vi "StopProcess.Do.vi"(8 "error in":errorcluster, 10 "State Variables":T5, 11 "gRPC Request":T1) -> (0 "error out":errorcluster, 2 "State Variables out":T5, 3 "gRPC Response":T3)   [LabVIEW 2025, in "bus_monitor_server_do.lvlib"]
doc: "Stop all XNET sessions (Incoming and Outgoing).\nStop Async StreamProcess.Main.vi."
uses:
  bus_monitor_server_do.lvlib
  bus_monitor_server/RPC Messages/ni_bus_monitor_api_StopProcessReply.ctl
  bus_monitor_server/bus_monitor_server.lvlib
  bus_monitor_server/RPC Messages/ni_bus_monitor_api_ErrorInfo.ctl
  Types/XNET.InitialSettings.ctl
  Types/StreamProcess.VIRef.ctl
  Types/StreamProcess.Refs.ctl
  Types/MainProcess.StateVariables.ctl
  bus_monitor_server/RPC Messages/ni_bus_monitor_api_StopProcessRequest.ctl
  bus_monitor_server/RPC Messages/ni_bus_monitor_api_Session.ctl
  bus_monitor_server/RPC Messages/ni_bus_monitor_api_FrameFilter.ctl
  bus_monitor_server/RPC Messages/ni_bus_monitor_api_DirectionFilter.ctl
  bus_monitor_server/RPC Messages/ni_bus_monitor_api_FilterInfo.ctl
  bus_monitor_server/RPC Messages/ni_bus_monitor_api_FdIsoMode.ctl
  bus_monitor_server/RPC Messages/ni_bus_monitor_api_Termination.ctl
  bus_monitor_server/RPC Messages/ni_bus_monitor_api_CanMode.ctl
  bus_monitor_server/RPC Messages/ni_bus_monitor_api_ConnectSettings.ctl
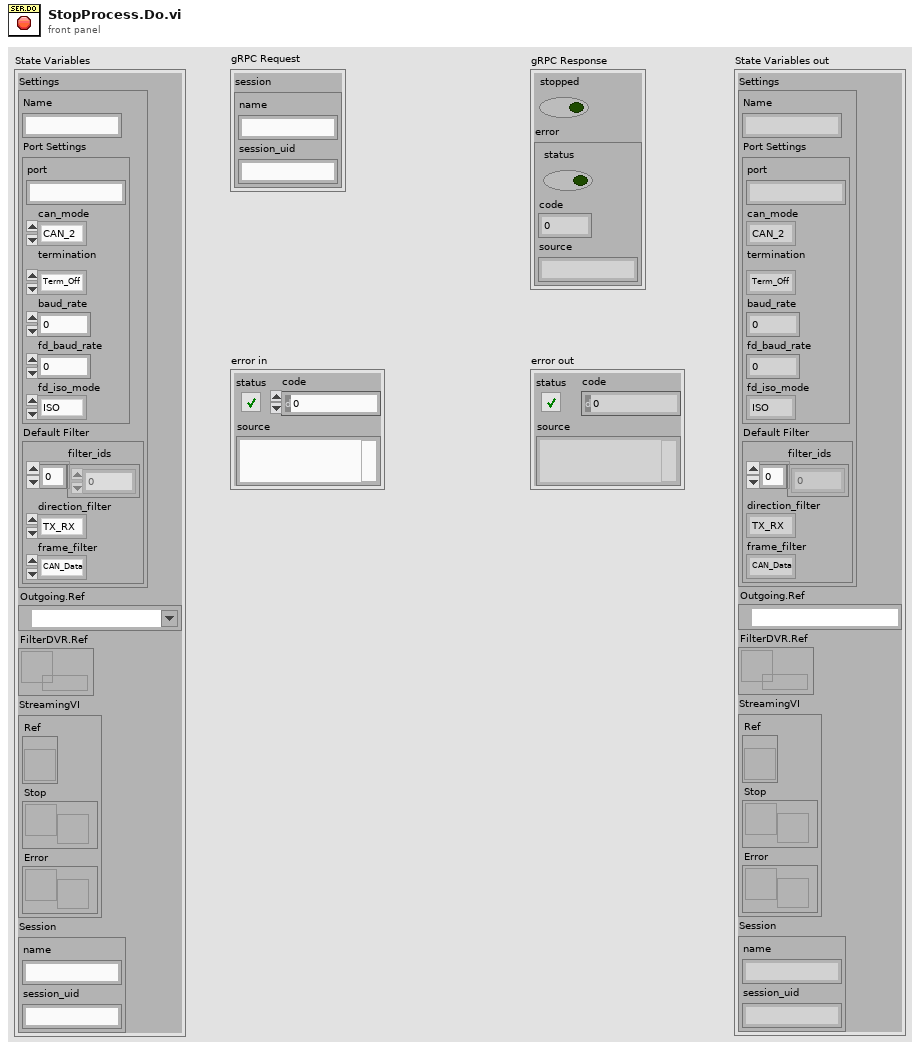
[diagram p1: front panel]
types:
  T1 = typedef "bus_monitor_server.lvlib/ni_bus_monitor_api_StopProcessRequest.ctl" = cluster{"session":T2}
  T2 = typedef "bus_monitor_server.lvlib/ni_bus_monitor_api_Session.ctl" = cluster{"name":string, "session_uid":string}
  T3 = typedef "bus_monitor_server.lvlib/ni_bus_monitor_api_StopProcessReply.ctl" = cluster{"stopped":bool, "error":T4}
  T4 = typedef "bus_monitor_server.lvlib/ni_bus_monitor_api_ErrorInfo.ctl" = errorcluster
  T5 = typedef "bus_monitor_server_do.lvlib/MainProcess.StateVariables.ctl" = cluster{"Settings":T6, "Outgoing.Ref":refnum<k21>, "FilterDVR.Ref":refnum<data-value>, "StreamingVI":T14, "Session":T2}
  T6 = typedef "bus_monitor_server_do.lvlib/XNET.InitialSettings.ctl" = cluster{"Name":string, "Port Settings":T7, "Default Filter":T11}
  T7 = typedef "bus_monitor_server.lvlib/ni_bus_monitor_api_ConnectSettings.ctl" = cluster{"port":string, "can_mode":T8, "termination":T9, "baud_rate":u64, "fd_baud_rate":u64, "fd_iso_mode":T10}
  T8 = typedef "bus_monitor_server.lvlib/ni_bus_monitor_api_CanMode.ctl" = enum32{"CAN_2", "CAN_FD", "CAN_FD_BRS"}
  T9 = typedef "bus_monitor_server.lvlib/ni_bus_monitor_api_Termination.ctl" = enum32{"Term_Off", "Term_On"}
  T10 = typedef "bus_monitor_server.lvlib/ni_bus_monitor_api_FdIsoMode.ctl" = enum32{"ISO", "Non_ISO", "ISO_Legacy"}
  T11 = typedef "bus_monitor_server.lvlib/ni_bus_monitor_api_FilterInfo.ctl" = cluster{"filter_ids":u32[], "direction_filter":T12, "frame_filter":T13}
  T12 = typedef "bus_monitor_server.lvlib/ni_bus_monitor_api_DirectionFilter.ctl" = enum32{"TX_RX", "RX", "TX"}
  T13 = typedef "bus_monitor_server.lvlib/ni_bus_monitor_api_FrameFilter.ctl" = enum32{"CAN_Data", "CAN_Remote", "CAN_Bus_Error", "CAN_2_Data", "CAN_FD_Data", "CAN_FD_BRS_Data", "J1939_Data", "Delay", "Log_Trigger", "Start_Trigger", "All"}
  T14 = typedef "bus_monitor_server_do.lvlib/StreamProcess.Refs.ctl" = cluster{"Ref":T15, "Stop":refnum<notifier>, "Error":refnum<notifier>}
  T15 = typedef "bus_monitor_server_do.lvlib/StreamProcess.VIRef.ctl" = refnum<vi>
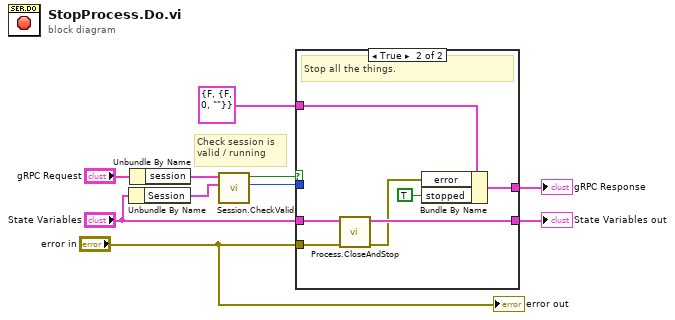
[diagram p0: block diagram]
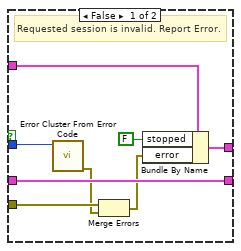
[diagram p2: hidden frame]
diagram:
  # "Check session is valid / running"
  n1 = Unbundle By Name("State Variables") -> ("Session"=w6:T2)
  n2 = Unbundle By Name("gRPC Request") -> ("session"=w5:T2)
  n3 = call "Session.CheckValid.vi"("Cached Session"=w6, "requested session"=w5) -> ("Error Code"=w1:i32, "Valid?"=w2:bool)  [unwired: 8 in]
  n4 = case shown="True" w2 {
    tunnel: [w15 w25] -> w10
    tunnel: [w16 w22] -> w9
    tunnel: "error in" -> [w13 w21]
    tunnel: "State Variables" -> [w15 w20]
    tunnel: T3 {"stopped"=FALSE, "error"={"status"=FALSE, "code"=0, "source"=""}} ("package_templatemessage") -> [w17 w19]
    tunnel: w1 -> [w14 _]
    frame False {
      # "Requested session is invalid. Report Error."
      n5 = call <vilib>:"Error Cluster From Error Code.vi"("error code (0)"=w14) -> ("error out"=w12:errorcluster)  [unwired: 8 in]
      n6 = Merge Errors(w13, w12) -> (w11:errorcluster)
      n7 = Bundle By Name(cluster=w17, "stopped"=FALSE, "error"=w11) -> (w16:T3)
    }
    frame True {
      # "Stop all the things."
      n8 = call "Process.CloseAndStop.vi"("error in"=w21, "State Variables"=w20) -> ("error out"=w23:errorcluster, "State Variables"=w25:T5)  [unwired: 8 in]
      n9 = Bundle By Name(cluster=w19, "error"=w23, "stopped"=TRUE) -> (w22:T3)
    }
  }
  "State Variables out" <- w10
  "gRPC Response" <- w9
  "error out" <- "error in"
